vi "CE GUI Recalculate.vi"(10 "CE measurement":T1={"Signal frequencies (Hz) T"=[1000.0], "Signal amplitudes (V) T"=[0.707], "Sampling frequencies (Hz) T"=[10000000.0], "Record lengths (multiples of periods) T"=[10000.0], "TWM data root directory"=path "", "TWM mreasurements directories"=[], "Calculate RMS from samples"=FALSE, "Algorithm to use"="TWM-WFFT", "Quantity to read"="TWM-WFFT", "Settle down after AC source change (s) T"=1.0, "Skip PJVS setup"=FALSE, "Measurement template file"=path "", "Row of START keyword T"=0, "Row of STOP keyword T"=0, "Measurement template line T"=[], "Switch position T"=[10000.0], "FR fit mat file T"=path "", "Recalculate-skip already calculated"=FALSE} {"Switch position T" format="%#_3p"; "Record lengths (multiples of periods) T" format="%#_3p"; "Sampling frequencies (Hz) T" format="%#_3p"; "Signal amplitudes (V) T" format="%#_3p"; "Signal frequencies (Hz) T" format="%#_3p"}, 11 "Common properties":T2={"Measurement status ref"=refnum, "TWM Status ref"=refnum, "Abort ref"=refnum, "Skip waiting ref"=refnum, "GNU Octave path"=path "C:/Program Files/GNU Octave/Octave-6.2.0/mingw64/bin", "TWM+QWTB path"=path "C:/Users/labina/Desktop/TWM-1.8.7.0-full/octprog", "lvlib path"=path "D:/martin/WAC/WACsw - github/control_software/Filter function meter/external libraries/GOLPI 0.7.3.1 source distribution LV 20.0 32 bit/lv_proc.dll", "TWM pipe"="\\\\.\\pipe\\TWM:server", "PJVS status ref"=refnum, "WAC path"=path ""}) -> (2 "CE measurement out":T1={"Signal frequencies (Hz) T"=[1000.0], "Signal amplitudes (V) T"=[0.707], "Sampling frequencies (Hz) T"=[10000000.0], "Record lengths (multiples of periods) T"=[10000.0], "TWM data root directory"=path "", "TWM mreasurements directories"=[], "Calculate RMS from samples"=FALSE, "Algorithm to use"="TWM-WFFT", "Quantity to read"="TWM-WFFT", "Settle down after AC source change (s) T"=1.0, "Skip PJVS setup"=FALSE, "Measurement template file"=path "", "Row of START keyword T"=0, "Row of STOP keyword T"=0, "Measurement template line T"=[], "Switch position T"=[10000.0], "FR fit mat file T"=path "", "Recalculate-skip already calculated"=FALSE} {"Switch position T" format="%#_3p"; "Record lengths (multiples of periods) T" format="%#_3p"; "Sampling frequencies (Hz) T" format="%#_3p"; "Signal amplitudes (V) T" format="%#_3p"; "Signal frequencies (Hz) T" format="%#_3p"})   [LabVIEW 2020]
doc: "GUI to setup and run (re)calculation of the data obtiained during the mesurement procedure used to estimate cable error."
uses:
  Utilities/Type definitions/Common properties.ctl
  CE Measurement/Type definitions/CE measurement.ctl
  <vilib>/Utility/NIReport.llb/Report Type.ctl
  <vilib>/Utility/error.llb/Error Cluster From Error Code.vi
  <vilib>/ErrorRing/Error Ring.xnode
  <vilib>/Utility/NIReport.llb/NI_report.lvclass
  external libraries/varilib/varilib.lvlib
  <vilib>/Utility/NIReport.llb/NI_ReportGenerationCore.lvlib
panel:
  out "template file":string
  in  "Abort":bool
  in  "skip calculated":bool caption="Skip already calculated (only rereads results)"
  out "Progress":i32(slide) min=0 max=266 scale=0.0..10.0
  out "gui_elements":refnum<vi>[](array[refnum])
  in  "OK":bool
  in  "cancel":bool
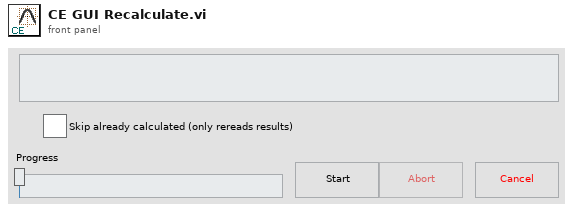
[diagram p1: front panel]
types:
  T1 = typedef "CE measurement.ctl" = cluster{"Signal frequencies (Hz) T":dbl[], "Signal amplitudes (V) T":dbl[], "Sampling frequencies (Hz) T":dbl[], "Record lengths (multiples of periods) T":dbl[], "TWM data root directory":path, "TWM mreasurements directories":path[], "Calculate RMS from samples":bool, "Algorithm to use":string, "Quantity to read":string, "Settle down after AC source change (s) T":dbl, "Skip PJVS setup":bool, "Measurement template file":path, "Row of START keyword T":i32, "Row of STOP keyword T":i32, "Measurement template line T":i32[], "Switch position T":dbl[], "FR fit mat file T":path, "Recalculate-skip already calculated":bool}
  T2 = typedef "Common properties.ctl" = cluster{"Measurement status ref":refnum<vi>, "TWM Status ref":refnum<vi>, "Abort ref":refnum<vi>, "Skip waiting ref":refnum<vi>, "GNU Octave path":path, "TWM+QWTB path":path, "lvlib path":path, "TWM pipe":string, "PJVS status ref":refnum<vi>, "WAC path":path}
  T3 = enum8{"Enabled", "Disabled", "Disabled and Grayed Out"}
  T4 = enum16{"maximized", "minimized", "normal", "no change"}
  T5 = typedef "NI_ReportGenerationCore.lvlib/Report Type.ctl" = enum16{"HTML", "Word", "Excel"}
  T6 = typedef "Type definitions to be saved.ctl" = cluster{"Common properties":T2, "AC Source":T7, "DC meter":T9, "CE measurement":T1, "FR measurement":T11, "FR template":T12, "CE template":T13, "PJVS":T14, "SS measurement":T18, "AC sync source":T7, "DG measurement":T19}
  T7 = typedef "AC Source.ctl" = cluster{"AC Source type":T8, "VISA":refnum<visa-resource-name>, "Ref. clock (Hz)":dbl, "status ref":refnum<vi>, "Fluke 57XX wideband output":bool, "Fluke 57XX ignore errors":bool, "Synchronization by AC signal":bool}
  T8 = typedef "AC Source type.ctl" = enum16{"Fluke 5XXX calibrator", "Tektronix AFG3000 series", "dummy", "Agilent 331xxA to 332xxA", "Agilent 335xxA to 336xxA"}
  T9 = typedef "DC meter.ctl" = cluster{"DC meter type":T10, "DC meter VISA":refnum<visa-resource-name>, "NPLC":dbl, "status ref":refnum<vi>}
  T10 = typedef "DC meter type.ctl" = enum16{"H/A/K 3458", "Fluke 8508A", "dummy", "Keithley 2182"}
  T11 = typedef "FR measuement.ctl" = cluster{"Measurement frequencies (Hz)":dbl[], "Sampling frequency (Hz)":dbl, "Signal amplitude (V)":dbl, "AC-DC settle time (s)":dbl, "Record length (multiples of period)":dbl[], "Measurement template file":path, "Row of START keyword":i32, "Row of STOP keyword":i32, "Calculate RMS from samples":bool, "AC-DC warm up time (s)":dbl, "Measurement template line":i32[], "DC meter readings No.":i32, "Algorithm":string, "Simultaneous measurement":bool, "Recalculate-skip already calculated":bool}
  T12 = typedef "FR template.ctl" = cluster{"Keywords column":i32, "Sig. freq. column":i32, "Rec. len. column":i32, "Meas. points. row min to read":i32, "Meas. points. row max to read":i32, "Properties column":i32, "Properties row start":i32, "Properties row end":i32, "Keyword START regexp":string, "Keyword STOP regexp":string, "HW data column":i32, "HW data row start":i32, "HW data row end":i32, "TIme and date column start":i32, "Digitizer value column start ":i32, "DC mean column start ":i32, "DC readings column start":i32}
  T13 = typedef "CE template.ctl" = cluster{"Keywords column":i32, "Sig. freq. column":i32, "Rec. len. column":i32, "Switch pos column":i32, "Meas. points. row min to read":i32, "Meas. points. row max to read":i32, "Properties column":i32, "Properties row start":i32, "Properties row end":i32, "Keyword START regexp":string, "Keyword STOP regexp":string, "HW data column":i32, "HW data row start":i32, "HW data row end":i32, "TIme and date column start":i32, "Digitizer value column start ":i32}
  T14 = typedef "PJVS.ctl" = cluster{"PJVS type":T15, "Status Refnum":refnum<vi>, "AC-supraVOLTcontrol":cluster{"IP address:port (0.0.0.0:0000)":string, "Timeouts":T16, "Simulation mode":bool, "Debug mode":bool}, "NPL bias source":cluster{"DataSocketCluster":T17}, "Manual PJVS":cluster{"PJVS frequency (Hz)":dbl, "Reference voltages (V)":dbl[], "File with PJVS voltages":path}, "VTT PJVS":cluster{"some VTT only property":string}}
  T15 = typedef "PJVS Type.ctl" = enum16{"AC-supraVOLTcontrol", "JV modified NPL bias control", "Manual PJVS", "VTT PJVS"}
  T16 = typedef "ACSVcontrol-driver.lvlib/Timeouts.ctl" = cluster{"TCP Read & Write (ms)":i32, "Sensors readout":i32, "PJVS setup":i32, "Nullmeter readout":i32, "Multiplexer setup":i32, "57XX setup":i32, "Generator setup":i32, "Synthesizer setup":i32, "Sampler readout":i32}
  T17 = typedef "DataSocketCluster external.ctl" = cluster{"Server Machine":string, "Client Machine":string, "Data":string, "TimeStamp":dbl, "Count":i32, "Target Process":string}
  T18 = typedef "SS measurement.ctl" = cluster{"Signal frequencies (Hz)":dbl[], "Signal amplitudes (V)":dbl[], "Sampling frequencies (Hz)":dbl[], "Record lengths (multiples of periods)":dbl[], "Calculate results":bool, "Algorithm":string, "TWM data directories":path[], "TWM data directories relative":path[], "Settle down after AC source change (s)":dbl, "PJVS frequencies (Hz)":dbl[], "PJVS reference voltages array of vector cluster":cluster{"PJVS reference voltages vector":dbl[]}[], "Requested PJVS steps":u32[], "Measure CE":bool, "Measure CE before":bool, "Measure CE after":bool, "Single point CE measurement":bool, "original CE template path":path, "new CE template path before SS":path, "new CE template path before SS relative":path, "new CE template path after SS":path, "new CE template path after SS relative":path, "original CE fit path":path, "new CE fit path before SS":path, "new CE fit path before SS relative":path, "new CE fit path after SS":path, "new CE fit path after SS relative":path, "Measure digitizer gain":bool, "Measure digitizer gain before":bool, "Measure digitizer gain after":bool, "Digitizer gain":dbl, "Data folder":path, "FR fit path":path, "new FR fit path relative":path, "Rs":i32, "Re":i32, "SS measurement info files":path[]}
  T19 = typedef "DG measurement.ctl" = cluster{"Sampling frequencies (Hz)":dbl[], "Requested PJVS frequencies (Hz)":dbl[], "Requested PJVS waveform amplitudes (V)":dbl[], "Record lengths (multiples of PJVS periods)":dbl[], "Requested PJVS steps":u32[], "Switch position":dbl, "Settle down after PJVS change (s)":dbl, "Rs":i32, "Re":i32, "Algorithm":string, "Calculate results":bool, "Data folder":path, "TWM data directories":path[], "TWM data directories relative":path[], "DG measurement info files":path[], "Set PJVS frequencies (Hz)":dbl[], "Set PJVS reference voltages array of vector cluster":cluster{"PJVS reference voltages vector":dbl[]}[], "Set PJVS steps":u32[]}
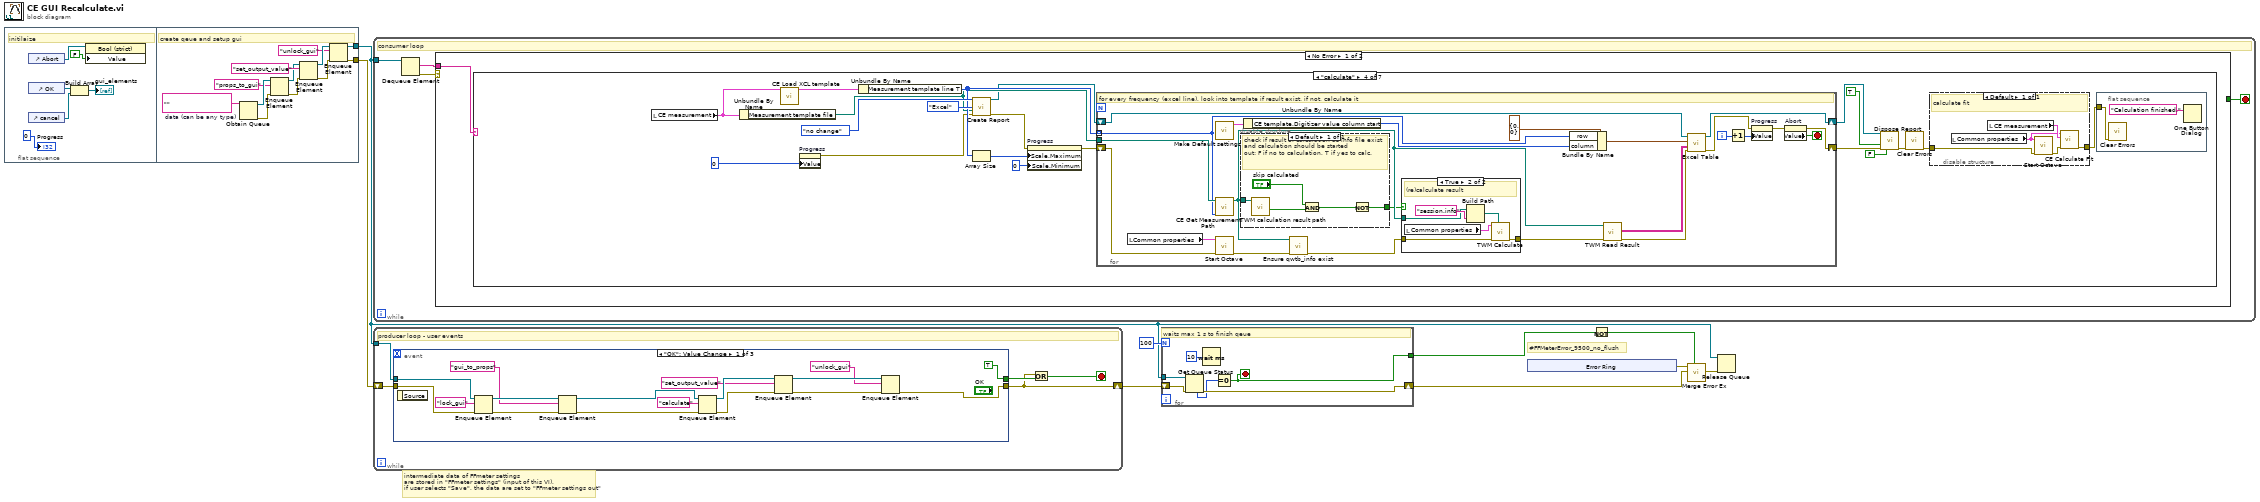
[diagram p0: block diagram]
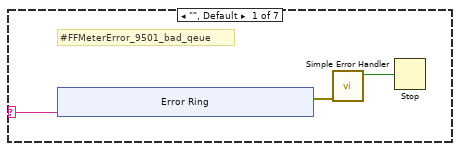
[diagram p2: hidden frame]
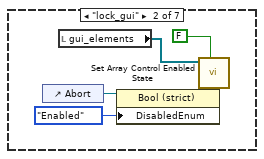
[diagram p3: hidden frame]
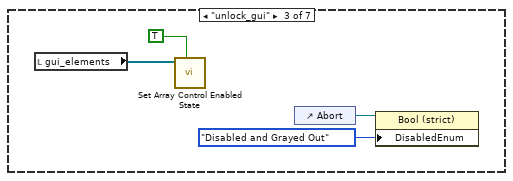
[diagram p4: hidden frame]
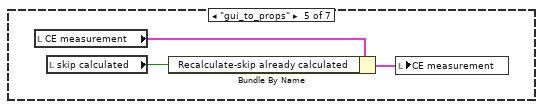
[diagram p6: hidden frame]
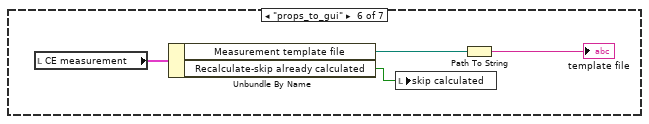
[diagram p7: hidden frame]
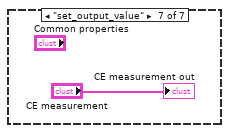
[diagram p8: hidden frame]
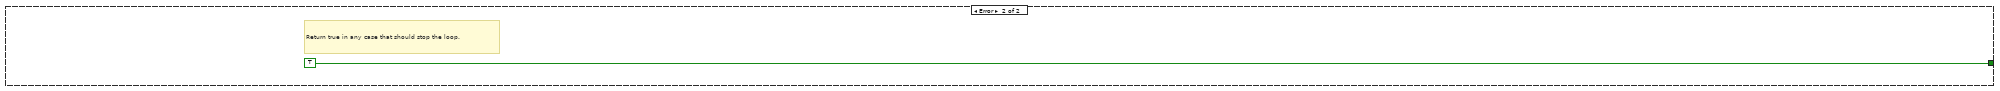
[diagram p9: hidden frame]
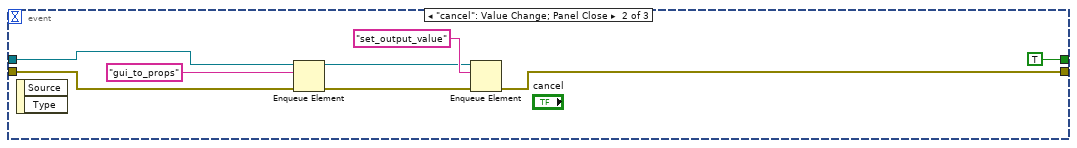
[diagram p10: hidden frame]
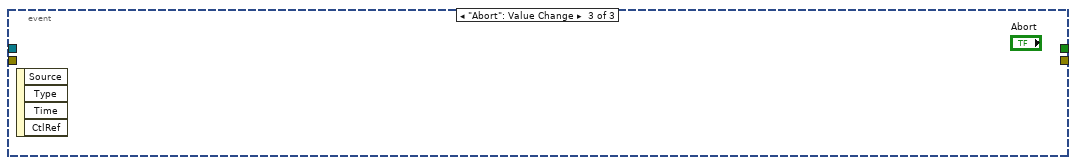
[diagram p11: hidden frame]
diagram:
  # "intermediate data of FFmeter settings\nare stored in \"FFmeter settings\" (input of this VI),\nif user selects \"Save\", the data are set to \"FFmeter settings out\""
  # "#FFMeterError_9500_no_flush"
  n1 = flat-sequence {
    tunnel: [w17] -> w2
    tunnel: [w18] -> w1
    frame #0 {
      # "initilaize"
      n2 = control-ref of="Abort"() -> (w11:refnum<vi>)
      n3 = control-ref of="OK"() -> (w15:refnum<vi>)
      n4 = control-ref of="cancel"() -> (w14:refnum<vi>)
      n5 = Build Array(w15, w14) -> (→"gui_elements":refnum<vi>[])
      n6 = property class="Bool (strict)"(reference=w11, "Value"=FALSE) -> ()  [unwired: 1 in, 2 out]
      "Progress" <- 0 ("Progress")
    }
    frame #1 {
      w26 = ""  # data (can be any type)
      # "create qeue and setup gui"
      n7 = Obtain Queue(element data type=w26) -> (queue out=w23:refnum<queue>, error out=w22:errorcluster)  [unwired: 4 in, 1 out]
      n8 = Enqueue Element(queue=w23, element="props_to_gui", error in (no error)=w22) -> (queue out=w24:refnum<queue>, error out=w25:errorcluster)  [unwired: 1 in, 1 out]
      n9 = Enqueue Element(queue=w24, element="set_output_value", error in (no error)=w25) -> (queue out=w20:refnum<queue>, error out=w19:errorcluster)  [unwired: 1 in, 1 out]
      n10 = Enqueue Element(queue=w20, element="unlock_gui", error in (no error)=w19) -> (queue out=w17:refnum<queue>, error out=w18:errorcluster)  [unwired: 1 in, 1 out]
    }
  }
  n11 = while {
    tunnel: w2 -> [w31]
    stop <- w28 stop-if-true
    # "consumer loop"
    n12 = Dequeue Element(queue=w31) -> (element=w29:string, error out=w30:errorcluster)  [unwired: 2 in, 2 out]
    n13 = case shown="No Error" w30 {
      tunnel: w29 -> [w32 _]
      tunnel: [_ TRUE] -> w28
      frame No Error {
        n14 = case shown="\"calculate\"" w32 {
          selector: w32 -> [w33 _ _ _ _ _ _]
          frame "", Default {
            # "#FFMeterError_9501_bad_qeue"
            n15 = xnode "Error Ring"("parameter 0"=w33) -> ("error out"=w35:errorcluster)
            n16 = call <vilib>:"Simple Error Handler.vi"("error in (no error)"=w35) -> ("error?"=w34:bool)  [unwired: 4 in, 4 out]
            n17 = Stop(stop? (T)=w34) -> ()
          }
          frame "lock_gui" {
            n18 = control-ref of="Abort"() -> (w44:refnum<vi>)
            n19 = local read "gui_elements"() -> (w46:refnum<vi>[])
            n20 = property class="Bool (strict)"(reference=w44, "DisabledEnum"=T3."Enabled" ("Disabled")) -> ()  [unwired: 1 in, 2 out]
            n21 = call "Set Array Control Enabled State.vi"("enabled (T)"=FALSE, "reference array in"=w46) -> ()  [unwired: 8 in, 2 out]
          }
          frame "unlock_gui" {
            n22 = local read "gui_elements"() -> (w50:refnum<vi>[])
            n23 = call "Set Array Control Enabled State.vi"("enabled (T)"=TRUE, "reference array in"=w50) -> ()  [unwired: 8 in, 2 out]
            n24 = control-ref of="Abort"() -> (w47:refnum<vi>)
            n25 = property class="Bool (strict)"(reference=w47, "DisabledEnum"=T3."Disabled and Grayed Out" ("Disabled")) -> ()  [unwired: 1 in, 2 out]
          }
          frame "calculate" {
            n26 = local read "CE measurement"() -> (w57:T1)
            n27 = Unbundle By Name(w57) -> ("Measurement template file"=w58:path)
            n28 = call "CE Load XCL template.vi"("CE measurement"=w57) -> ("CE measurement out"=w56:T1)  [unwired: 9 in, 1 out]
            n29 = property on="Progress" class="Slide (strict)"("Value"=0 ("Progress")) -> (error out=w66:errorcluster)  [unwired: 2 in, 1 out]
            n30 = Unbundle By Name(w56) -> ("Measurement template line T"=w68:i32[])
            n31 = Array Size(array=w68) -> (size(s)=w67:i32)
            n32 = call <vilib>:"Create Report.vi"("window state (normal)"=T4."no change", "report type"=Report_Type."Excel", "template (empty)"=w58, "error in (no error)"=w66) -> ("report out"=w54:refnum<class "NI_report.lvclass">, "error out"=w55:errorcluster)  [unwired: 10 in]
            n33 = property on="Progress" class="Slide (strict)"(error in=w55, "Scale.Maximum"=w67, "Scale.Minimum"=0 ("Data Entry Limits:Minimum")) -> (error out=w64:errorcluster)  [unwired: 1 in, 1 out]
            n34 = for {
              tunnel: w68 -> [w87] mode=indexing
              shift-right: [w89] -> w61
              shift-left: w64 -> [w98]
              shift-right: [w93] -> w62
              shift-left: w54 -> [w99]
              tunnel: w58 -> [w88]
              i -> [w100]
              stop <- w90 stop-if-true
              # "for every frequency (excel line), look into template if result exist. if not, calculate it"
              n35 = local read "Common properties"() -> (w78:T2)
              n36 = call "Make Default settings.vi"() -> ("TD to be saved"=w80:T6)  [unwired: 11 in]
              n37 = call "CE Get Measurement Path.vi"("Template line"=w87, "Measurement template file"=w88) -> ("Measurement path"=w86:path)  [unwired: 8 in, 1 out]
              n38 = call "Start Octave.vi"("error in (no error)"=w98, "Common properties"=w78) -> ("error out"=w96:errorcluster)  [unwired: 9 in]
              n39 = disable-structure shown="Default" {
                disable-tunnel: w86 -> [w105]
                disable-tunnel: [w101] -> w85
                frame Enabled {
                  # "check if result of calculation as info file exist\nand calculation should be started\nout: F if no to calculation, T if yes to calc."
                  n40 = call "TWM calculation result path.vi"("Measurement path"=w105) -> ("file exists?"=w103:bool)  [unwired: 9 in, 1 out]
                  n41 = Compound Arithmetic op=AND("skip calculated", w103) -> (w102:bool)
                  n42 = Not(x=w102) -> (.not. x?=w101:bool)
                }
              }
              n43 = Unbundle By Name(w80) -> ("CE template.Digitizer value column start"=w79:i32)
              n44 = call "Ensure qwtb_info exist.vi"("error in"=w96, "Measurement path"=w86) -> ("error out"=w95:errorcluster)  [unwired: 9 in]
              n45 = case shown="True" w85 {
                tunnel: w95 -> [w106 w112]
                tunnel: [w106 w111] -> w92
                tunnel: w86 -> [_ w109]
                frame False {
                  # "no calculation"
                }
                frame True {
                  # "(re)calculate result"
                  n46 = local read "Common properties"() -> (w107:T2)
                  n47 = Build Path(base path=w109, name or relative path="session.info") -> (appended path=w108:path)
                  n48 = call "TWM Calculate.vi"("session info path"=w108, "error in (no error)"=w112, "Common properties"=w107) -> ("error out"=w111:errorcluster)  [unwired: 8 in]
                }
              }
              n49 = Bundle By Name(cluster=cluster{"row":i32, "column":i32} {"row"=0, "column"=0} ("start (0, 0)"), "row"=w87, "column"=w79) -> (w83:cluster{"row":i32, "column":i32})
              n50 = call "TWM Read Result.vi"("error in (no error)"=w92, "Measurement path"=w86) -> ("error out"=w82:errorcluster, "Result (val, unc)"=w81:string[][])  [unwired: 8 in]
              n51 = call "Excel Table.vi"("error in (no error)"=w82, "table"=w81, "start (0, 0)"=w83, "report in"=w99) -> ("error out"=w94:errorcluster, "report out"=w93:refnum<class "NI_report.lvclass">)  [unwired: 6 in]
              n52 = Increment(x=w100) -> (x+1=w97:i32)
              n53 = property on="Progress" class="Slide (strict)"(error in=w94, "Value"=w97) -> (error out=w91:errorcluster)  [unwired: 1 in, 1 out]
              n54 = property on="Abort" class="Bool (strict)"(error in=w91) -> (error out=w89:errorcluster, "Value"=w90:bool)  [unwired: 1 in, 1 out]
            }
            n55 = call-dynamic "Dispose Report.vi"("report in"=w62, "save changes? (F)"=TRUE, "error in (no error)"=w61, "close report? (T)"=FALSE) -> ("error out"=w53:errorcluster)  [unwired: 11 in]
            n56 = call <vilib>:"Clear Errors.vi"("error in (no error)"=w53) -> ("error out"=w52:errorcluster)  [unwired: 5 in, 1 out]
            n57 = disable-structure shown="Default" {
              disable-tunnel: w52 -> [w74]
              disable-tunnel: [w72] -> w51
              frame Enabled {
                # "calculate fit"
                n58 = local read "Common properties"() -> (w71:T2)
                n59 = local read "CE measurement"() -> (w73:T1)
                n60 = call "Start Octave.vi"("error in (no error)"=w74, "Common properties"=w71) -> ("error out"=w75:errorcluster)  [unwired: 9 in]
                n61 = call "CE Calculate Fit.vi"("error in (no error)"=w75, "CE measurement"=w73, "Common properties"=w71) -> ("error out"=w72:errorcluster)  [unwired: 8 in]
              }
            }
            n62 = flat-sequence {
              tunnel: w51 -> [w76]
              frame #0 {
                n63 = call <vilib>:"Clear Errors.vi"("error in (no error)"=w76) -> ()  [unwired: 5 in, 2 out]
                n64 = One Button Dialog(message="Calculation finished.") -> ()  [unwired: 1 in, 1 out]
              }
            }
          }
          frame "gui_to_props" {
            n65 = local read "CE measurement"() -> (w115:T1)
            n66 = local read "skip calculated"() -> (w114:bool)
            n67 = Bundle By Name(cluster=w115, "Recalculate-skip already calculated"=w114) -> (w113:T1)
            n68 = local write "CE measurement"(w113) -> ()
          }
          frame "props_to_gui" {
            n69 = local read "CE measurement"() -> (w118:T1)
            n70 = Unbundle By Name(w118) -> ("Measurement template file"=w116:path, "Recalculate-skip already calculated"=w117:bool)
            n71 = local write "skip calculated"(w117) -> ()
            n72 = Path To String(path=w116) -> (string=→"template file":string)
          }
          frame "set_output_value" {
            "CE measurement out" <- "CE measurement"
          }
        }
      }
      frame Error {
        # "Return true in any case that should stop the loop."
      }
    }
  }
  n73 = while {
    shift-right: [w122] -> w5
    shift-left: w1 -> [w125]
    tunnel: w2 -> [w126]
    stop <- w123 stop-if-true
    # "producer loop - user events"
    n74 = event shown="[0] \"OK\": Value Change" {
      selector: _ -> [_ _ _]
      dyn-events: _ -> [_ _ _]
      timeout: _ -> [_ _ _]
      tunnel: w126 -> [w141 w145 _]
      tunnel: w125 -> [w140 w148 _]
      tunnel: [w132 w149 _] -> w122
      tunnel: [TRUE ("cancel") TRUE ("cancel") _] -> w124
      event "OK": Value Change {
        n75 = event-data() -> ()  [unwired: 1 in, 1 out]
        n76 = Enqueue Element(queue=w141, element="lock_gui", error in (no error)=w140) -> (queue out=w138:refnum<queue>, error out=w139:errorcluster)  [unwired: 1 in, 1 out]
        n77 = Enqueue Element(queue=w138, element="gui_to_props", error in (no error)=w139) -> (queue out=w130:refnum<queue>, error out=w129:errorcluster)  [unwired: 1 in, 1 out]
        n78 = Enqueue Element(queue=w130, element="calculate", error in (no error)=w129) -> (queue out=w135:refnum<queue>, error out=w136:errorcluster)  [unwired: 1 in, 1 out]
        n79 = Enqueue Element(queue=w135, element="set_output_value", error in (no error)=w136) -> (queue out=w131:refnum<queue>, error out=w133:errorcluster)  [unwired: 1 in, 1 out]
        n80 = Enqueue Element(queue=w131, element="unlock_gui", error in (no error)=w133) -> (error out=w132:errorcluster)  [unwired: 1 in, 2 out]
      }
      event "cancel": Value Change; Panel Close {
        n81 = event-data() -> ()  [unwired: 1 in, 2 out]
        n82 = Enqueue Element(queue=w145, element="gui_to_props", error in (no error)=w148) -> (queue out=w146:refnum<queue>, error out=w147:errorcluster)  [unwired: 1 in, 1 out]
        n83 = Enqueue Element(queue=w146, element="set_output_value", error in (no error)=w147) -> (error out=w149:errorcluster)  [unwired: 1 in, 2 out]
      }
      event "Abort": Value Change {
        n84 = event-data() -> ()  [unwired: 1 in, 4 out]
      }
    }
    n85 = Or(x=w122, y=w124) -> (x .or. y?=w123:bool)
  }
  n86 = for {
    N: 100 -> [_]
    tunnel: w2 -> [w157]
    shift-right: [w155] -> w6
    shift-left: w5 -> [w156]
    tunnel: [w152] -> w3
    stop <- w152 stop-if-true
    # "waits max 1 s to finish qeue"
    n87 = Get Queue Status(queue=w157, error in (no error)=w156) -> (error out=w155:errorcluster, # elements in queue=w153:i32)  [unwired: 1 in, 6 out]
    n88 = Wait (ms)(milliseconds to wait=u32 10) -> ()  [unwired: 1 out]
    n89 = Equal To 0?(x=w153) -> (x = 0?=w152:bool)
  }
  n90 = xnode "Error Ring"() -> ("error out"=w7:errorcluster)
  n91 = Not(x=w3) -> (.not. x?=w8:bool)
  n92 = call "Merge Error Ex.vi"("Is error? (False)"=w8, "main error in (no error)"=w6, "second error in"=w7) -> ("error out"=w4:errorcluster)  [unwired: 8 in]
  n93 = Release Queue(queue=w2, error in (no error)=w4) -> ()  [unwired: 1 in, 3 out]
